vi "Scan2graph.vi"() -> ()   [LabVIEW 2013]
panel:
  in  "Lancer man. c++":bool
  out "Affichage des erreurs":string
  out "Affichage du code":string
  in  "Valider choix fichier":bool
  in  "Passer à la suite...":bool
  in  "Zoom":dbl(slide) scale=1.0..10.0
  in  "Selectionner une image *.png":path
  out "Image à retravailler":picture
  # "0:"
  # "Run VI"
  # "1:"
  # "3:"
  # "4:"
  # "5:"
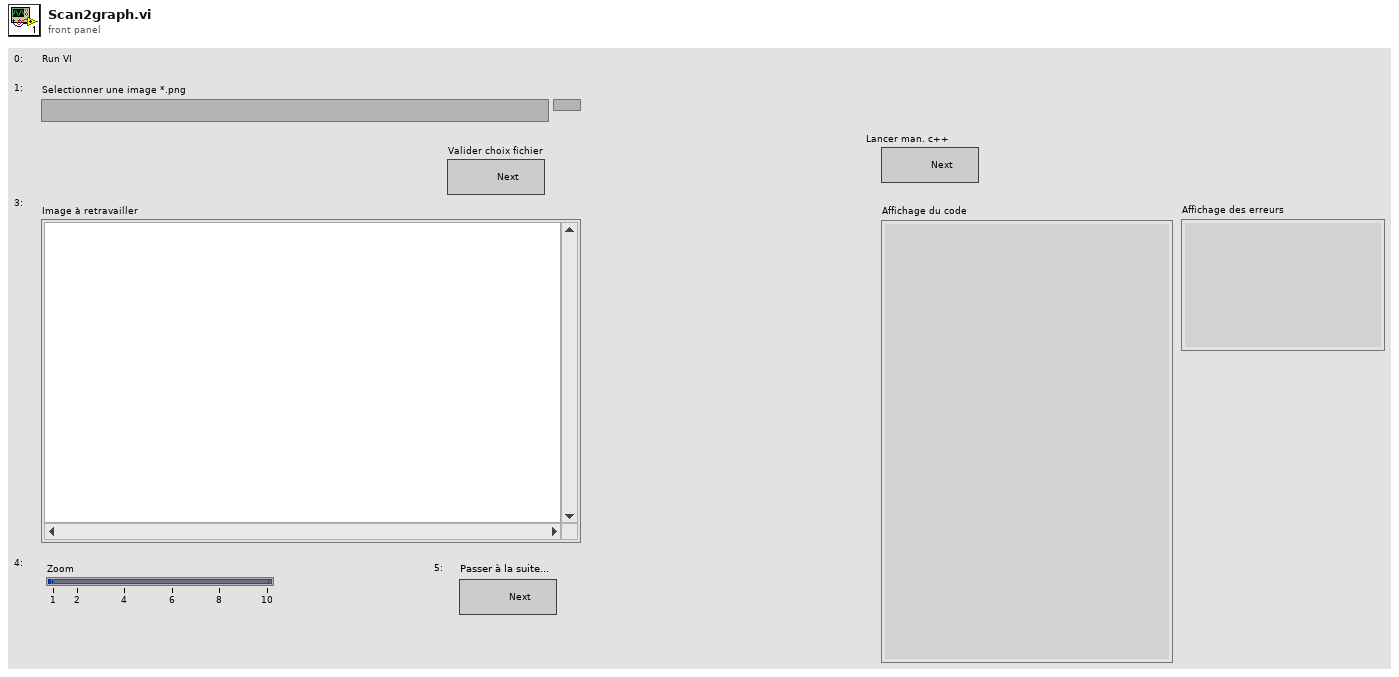
[diagram p1: front panel]
types:
  T1 = typedef "imagedata.ctl" = cluster{"image type":i32, "image depth":i32, "image":u8[], "mask":u8[], "colors":u32[], "Rectangle":cluster{"left":i16, "top":i16, "right":i16, "bottom":i16}}
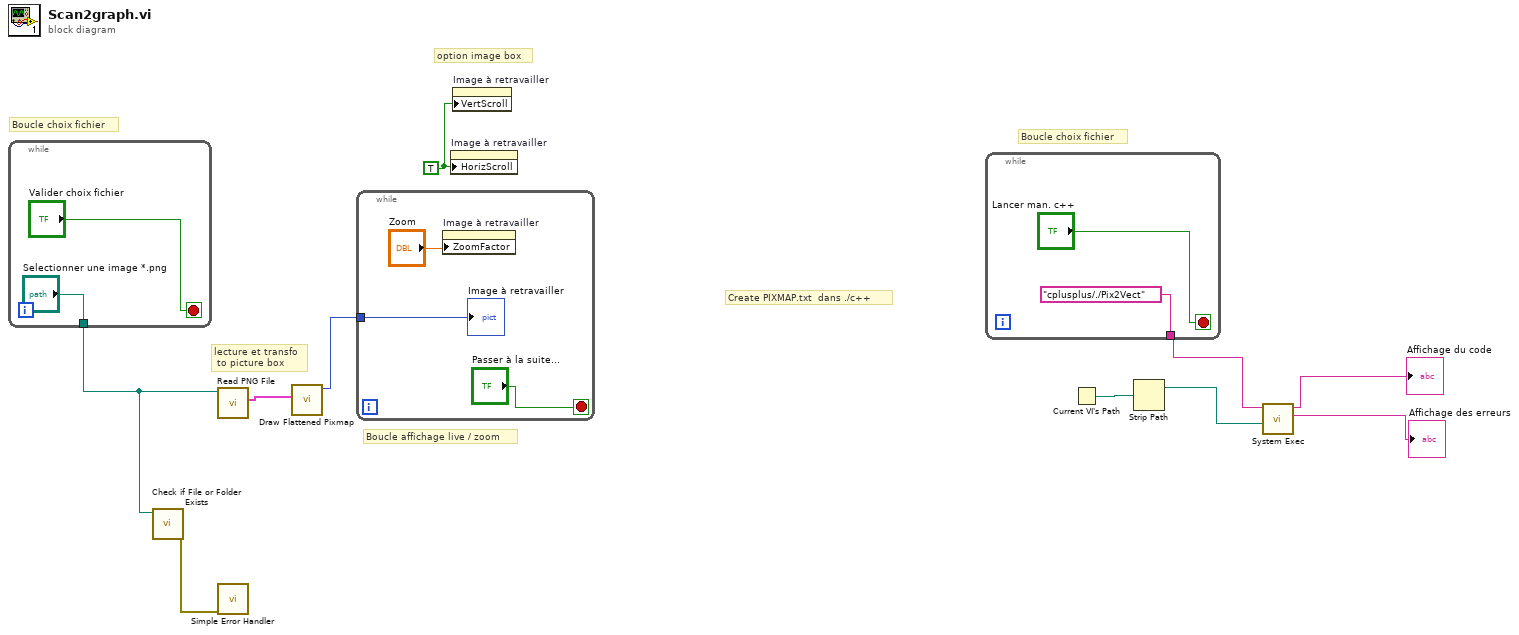
[diagram p0: block diagram]
diagram:
  w9 = TRUE ("Horizontal Scrollbar Visible")
  # "Boucle choix fichier"
  # "Create PIXMAP.txt  dans ./c++"
  # "lecture et transfo\n to picture box"
  # "option image box"
  # "Boucle affichage live / zoom"
  # "Boucle choix fichier"
  n1 = while {
    tunnel: ["Selectionner une image *.png"] -> w8
    stop <- "Valider choix fichier" stop-if-true
  }
  n2 = call <vilib>:"Check if File or Folder Exists.vi"("path"=w8) -> ("error out"=w10:errorcluster)  [unwired: 8 in, 2 out]
  n3 = call <vilib>:"Read PNG File.vi"("path to PNG file"=w8) -> ("image data"=w6:T1)  [unwired: 8 in, 2 out]
  n4 = call <vilib>:"Simple Error Handler.vi"("error in (no error)"=w10) -> ()  [unwired: 4 in, 5 out]
  n5 = call <vilib>:"Draw Flattened Pixmap.vi"("image data"=w6) -> ("new picture"=w7:picture)  [unwired: 8 in]
  n6 = while {
    tunnel: w7 -> [w14]
    stop <- "Passer à la suite..." stop-if-true
    n7 = property on="Image à retravailler" class="Pict"("ZoomFactor"="Zoom") -> ()  [unwired: 2 in, 2 out]
    "Image à retravailler" <- w14
  }
  n8 = property on="Image à retravailler" class="Pict"("HorizScroll"=w9) -> ()  [unwired: 2 in, 2 out]
  n9 = property on="Image à retravailler" class="Pict"("VertScroll"=w9) -> ()  [unwired: 2 in, 2 out]
  n10 = while {
    tunnel: ["cplusplus/./Pix2Vect"] -> w1
    stop <- "Lancer man. c++" stop-if-true
  }
  n11 = Current VI's Path() -> (path=w3:path)
  n12 = Strip Path(path=w3) -> (stripped path=w2:path)  [unwired: 1 out]
  n13 = call <vilib>:"System Exec.vi"("working directory"=w2, "command line"=w1) -> ("standard error"=→"Affichage des erreurs":string, "standard output"=→"Affichage du code":string)  [unwired: 6 in, 2 out]
